vi "getStopMechanism.vi"(8 "error in (no error)":errorcluster, 11 "ExampleTask_StopNotifier in":refnum<class "Task_BoolStopNotifier.lvclass">) -> (0 "error out":errorcluster, 2 "stopMechanism":refnum<class "ITaskStopMechanism.lvclass">, 3 "ExampleTask_StopNotifier out":refnum<class "Task_BoolStopNotifier.lvclass">)   [LabVIEW 2023, in "Task_BoolStopNotifier.lvclass"]
doc: "Returns the stop mechanism type used by the task."
uses:
  Task_BoolStopNotifier.lvclass
  ITaskStopMechanism/ITaskStopMechanism.lvclass
  BoolNotifierStopMech/BoolNotifierStopMechanism.lvclass
  C:/projects/TLC_Daemon/source/ITaskStopMechanism/ITaskStopMechanism.lvclass
  Task_BoolStopNotifier.lvclass/Task_BoolStopNotifier.ctl
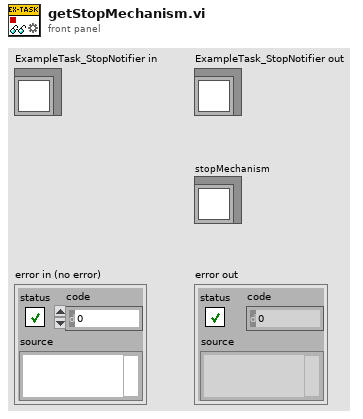
[diagram p1: front panel]
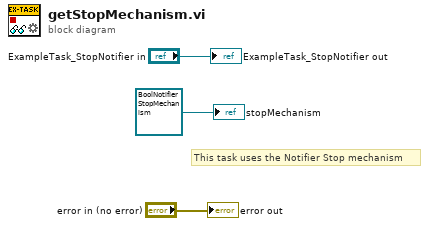
[diagram p0: block diagram]
diagram:
  # "This task uses the Notifier Stop mechanism"
  "error out" <- "error in (no error)"
  "ExampleTask_StopNotifier out" <- "ExampleTask_StopNotifier in"
  "stopMechanism" <- refnum<class "BoolNotifierStopMechanism.lvclass"> refnum ("TLC_Daemon.lvlib:NotifierStopMechanism.lvclass")
